vi "While_loop_with_timer_exit.vi"() -> ()   [LabVIEW 2021]
panel:
  out "Iteration":i32
  in  "Seconds":dbl=10.0 format="%.2f"
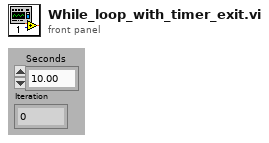
[diagram p1: front panel]
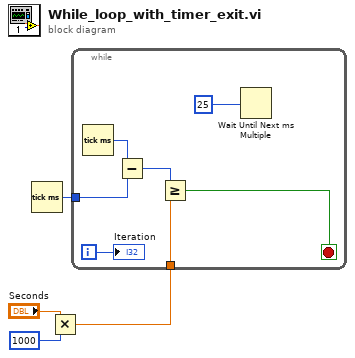
[diagram p0: block diagram]
diagram:
  n1 = Tick Count (ms)() -> (millisecond timer value=w4:u32)
  n2 = Multiply(x="Seconds", y=1000) -> (x*y=w1:dbl)
  n3 = while {
    tunnel: w4 -> [w10]
    tunnel: w1 -> [w8]
    i -> [w5]
    stop <- w7 stop-if-true
    n4 = Tick Count (ms)() -> (millisecond timer value=w11:u32)
    n5 = Subtract(x=w11, y=w10) -> (x-y=w9:u32)
    n6 = Greater Or Equal?(x=w9, y=w8) -> (x >= y?=w7:bool)
    n7 = Wait Until Next ms Multiple(millisecond multiple=25) -> ()  [unwired: 1 out]
    "Iteration" <- w5
  }
